vi "Robot_Main-backup.vi"() -> ()   [LabVIEW 2013]
uses:
  PolarCoordTdef.ctl
  StopTDef.ctl
  GainsTDef.ctl
  Support VIs/setpointCluster.ctl
  <vilib>/robotics/Starter Kit/2.0/9632 Host Interface/NI_Robotics_Starter Kit Host_9632_2.0.lvclass
  Support VIs/robotStop.vi
  Support VIs/gainsGlobalBot.vi
  Support VIs/setpointsGlobal.vi
  <vilib>/robotics/Starter Kit/Host Interface/NI_Robotics_Starter Kit Host.lvclass
panel:
  out "Kd-Arg":dbl
  out "Kc-Arg":dbl
  out "Kd-Mod":dbl
  out "Kc-Mod":dbl
  out "Modulus Setpoint Read":dbl
  out "Argument Setpoint Read":dbl
  out "Mod":dbl
  out "Arg":dbl
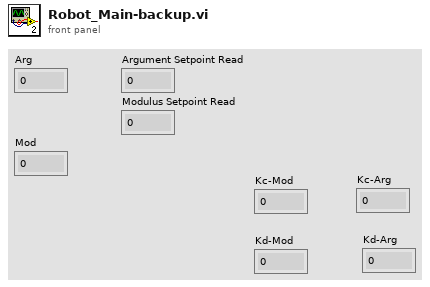
[diagram p1: front panel]
types:
  T1 = typedef "PolarCoordTdef.ctl" = cluster{"Argument":dbl, "Modulus":dbl, "trackedState":bool}
  T2 = typedef "StopTDef.ctl" = cluster{"stop":bool}
  T3 = typedef "GainsTDef.ctl" = cluster{"Kc-Modulus":dbl, "Kd-Modulus":dbl, "Kc-Argument":dbl, "Kd-Argument":dbl}
  T4 = typedef "setpointCluster.ctl" = cluster{"Modulus Setpoint":dbl, "Argument Setpoint":dbl}
  T5 = typedef "Messages.ctl" = cluster{"message data":variant, "message type":enum16{"Stop", "PolarCoordinates", "Gains", "Setpoints"}}
  T6 = cluster{"Kc-Modulus":dbl, "Kd-Modulus":dbl, "Kc-Argument":dbl, "Kd-Argument":dbl}
  T7 = enum16{"Stop", "PolarCoordinates", "Gains", "Setpoints"}
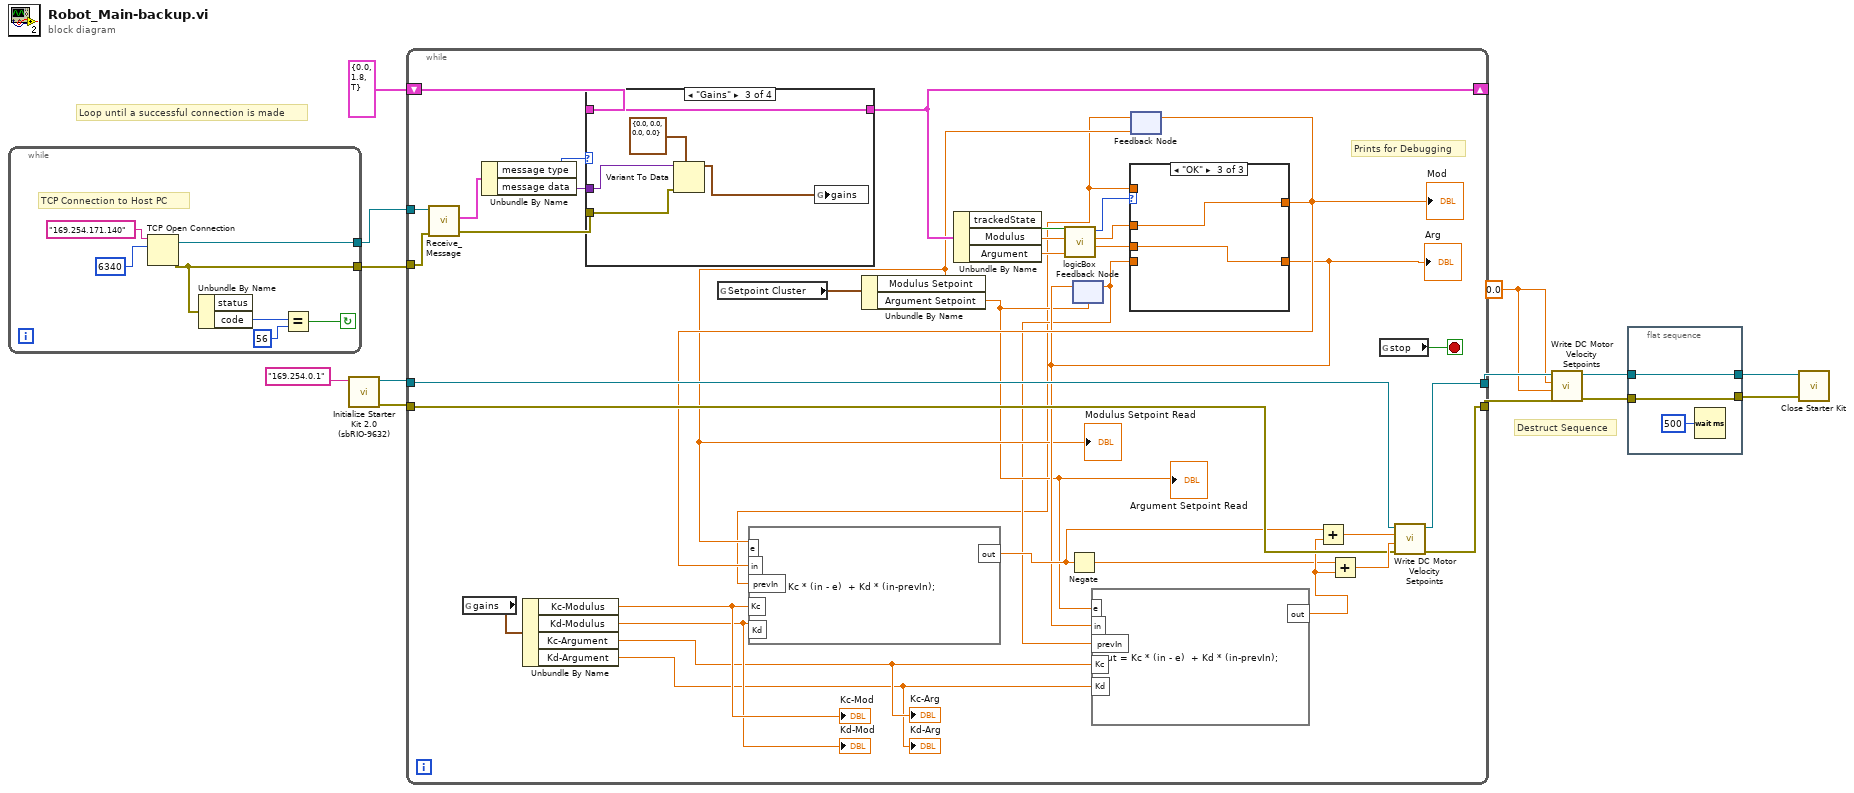
[diagram p0: block diagram]
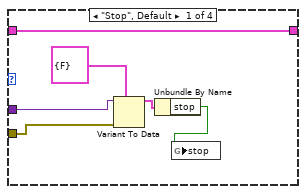
[diagram p2: hidden frame]
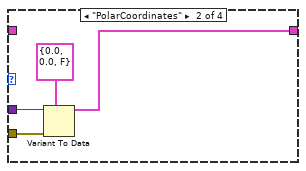
[diagram p3: hidden frame]
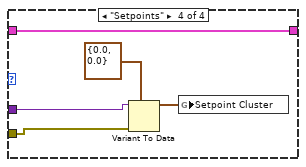
[diagram p4: hidden frame]
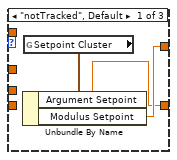
[diagram p5: hidden frame]
diagram:
  w9 = 0.0
  # "Loop until a successful connection is made"
  # "Destruct Sequence"
  n1 = while {
    tunnel: [w20] -> w2
    tunnel: [w17] -> w3
    stop <- w14 continue-if-true
    # "TCP Connection to Host PC"
    n2 = TCP Open Connection(address="169.254.171.140", remote port or service name=u16 6340) -> (connection ID=w20:refnum<k5>, error out=w17:errorcluster)  [unwired: 3 in]
    n3 = Unbundle By Name(w17) -> ("code"=w16:i32)  [unwired: 1 out]
    n4 = Equal?(x=w16, y=56) -> (x = y?=w14:bool)
  }
  n5 = call <vilib>:"Initialize Starter Kit 2.0 (sbRIO-9632).vi"("IP address (\"\")"="169.254.0.1" ("IP address (\"\")")) -> ("error out"=w12:errorcluster, "FPGA starter kit host 2.0 out"=w13:refnum<class "NI_Robotics_Starter Kit Host_9632_2.0.lvclass">)  [unwired: 9 in]
  n6 = while {
    tunnel: w13 -> [w54]
    tunnel: w12 -> [w53]
    tunnel: w3 -> [w42]
    tunnel: [w52] -> w11
    tunnel: [w51] -> w10
    tunnel: w2 -> [w43]
    shift-right: [w39] -> _
    shift-left: T1 {"Argument"=0.0, "Modulus"=1.8, "trackedState"=TRUE} ("Polar Coord") -> [w38]
    stop <- w41 stop-if-true
    # "Prints for Debugging"
    n7 = call "Receive_Message.vi"("error in (no error)"=w42, "connection ID IN"=w43) -> ("error out (no error)"=w44:errorcluster, "msg OUT"=w47:T5)  [unwired: 7 in, 1 out]
    n8 = global read "gainsGlobalBot.vi" "gains"() -> (w40:T6)
    n9 = Unbundle By Name(w47) -> ("message type"=w46:T7, "message data"=w45:variant)
    n10 = Unbundle By Name(w40) -> ("Kc-Modulus"=w24:dbl, "Kd-Modulus"=w23:dbl, "Kc-Argument"=w22:dbl, "Kd-Argument"=w21:dbl)
    "Kc-Mod" <- w24
    "Kd-Mod" <- w23
    "Kc-Arg" <- w22
    "Kd-Arg" <- w21
    n11 = case shown="\"Gains\"" w46 {
      tunnel: w45 -> [w61 w65 w70 w75]
      tunnel: w44 -> [w60 w64 w69 w74]
      tunnel: [w57 w63 w67 w72] -> w39
      tunnel: w38 -> [w57 _ w67 w72]
      frame "Stop", Default {
        n12 = Variant To Data(error in=w60, type=T2 {"stop"=FALSE}, Variant=w61) -> (data=w59:T2)  [unwired: 1 out]
        n13 = Unbundle By Name(w59) -> ("stop"=w58:bool)
        n14 = global write "robotStop.vi" "stop"(w58) -> ()
      }
      frame "PolarCoordinates" {
        n15 = Variant To Data(error in=w64, type=T1 {"Argument"=0.0, "Modulus"=0.0, "trackedState"=FALSE} ("Polar Coord"), Variant=w65) -> (data=w63:T1)  [unwired: 1 out]
      }
      frame "Gains" {
        n16 = Variant To Data(error in=w69, type=T3 {"Kc-Modulus"=0.0, "Kd-Modulus"=0.0, "Kc-Argument"=0.0, "Kd-Argument"=0.0} ("GainsCluster"), Variant=w70) -> (data=w68:T3)  [unwired: 1 out]
        n17 = global write "gainsGlobalBot.vi" "gains"(w68) -> ()
      }
      frame "Setpoints" {
        n18 = Variant To Data(error in=w74, type=T4 {"Modulus Setpoint"=0.0, "Argument Setpoint"=0.0} ("Setpoint Cluster"), Variant=w75) -> (data=w73:T4)  [unwired: 1 out]
        n19 = global write "setpointsGlobal.vi" "Setpoint Cluster"(w73) -> ()
      }
    }
    n20 = global read "setpointsGlobal.vi" "Setpoint Cluster"() -> (w29:T4)
    n21 = Unbundle By Name(w29) -> ("Modulus Setpoint"=w28:dbl, "Argument Setpoint"=w27:dbl)
    "Argument Setpoint Read" <- w27
    "Modulus Setpoint Read" <- w28
    n22 = Unbundle By Name(w39) -> ("trackedState"=w37:bool, "Modulus"=w36:dbl, "Argument"=w35:dbl)
    n23 = call "logicBox.vi"("Arg"=w35, "Mod"=w36, "TrackState"=w37) -> ("Arg"=w32:dbl, "Mod"=w33:dbl, "State"=w34:enum16{"notTracked", "NullMessage", "OK"})  [unwired: 6 in]
    n24 = feedback #1(w27) -> (w26:dbl)
    n25 = feedback #2(w28) -> (w25:dbl)
    n26 = case shown="\"OK\"" w34 {
      tunnel: [w77 w80 w82] -> w30
      tunnel: [w78 w81 w83] -> w31
      tunnel: w33 -> [_ _ w83]
      tunnel: w32 -> [_ _ w82]
      tunnel: w25 -> [_ w81 _]
      tunnel: w26 -> [_ w80 _]
      frame "notTracked", Default {
        n27 = global read "setpointsGlobal.vi" "Setpoint Cluster"() -> (w79:T4)
        n28 = Unbundle By Name(w79) -> ("Argument Setpoint"=w77:dbl, "Modulus Setpoint"=w78:dbl)
      }
      frame "NullMessage" {
      }
      frame "OK" {
      }
    }
    "Arg" <- w30
    "Mod" <- w31
    n29 = formula code="out = Kc * (in - e)  + Kd * (in-prevIn);"("e"=w28, "in"=w31, "prevIn"=w25, "Kc"=w24, "Kd"=w23) -> ("out"=w48:dbl)
    n30 = Negate(x=w48) -> (-x=w49:dbl)
    n31 = feedback-in #1(w30) -> ()
    n32 = formula code="out = Kc * (in - e)  + Kd * (in-prevIn);"("e"=w27, "in"=w30, "prevIn"=w26, "Kc"=w22, "Kd"=w21) -> ("out"=w50:dbl)
    n33 = feedback-in #2(w31) -> ()
    n34 = Add(x=w48, y=w50) -> (x+y=w56:dbl)
    n35 = Add(x=w49, y=w50) -> (x+y=w55:dbl)
    n36 = global read "robotStop.vi" "stop"() -> (w41:bool)
    n37 = call <vilib>:"Write DC Motor Velocity Setpoints.vi"("error in (no error)"=w53, "right motor ccw velocity (rad/s)"=w55, "left motor ccw velocity (rad/s)"=w56, "starter kit host in"=w54) -> ("error out"=w51:errorcluster, "starter kit host out"=w52:refnum<class "NI_Robotics_Starter Kit Host_9632_2.0.lvclass">)  [unwired: 6 in]
  }
  n38 = call <vilib>:"Write DC Motor Velocity Setpoints.vi"("error in (no error)"=w10, "right motor ccw velocity (rad/s)"=w9, "left motor ccw velocity (rad/s)"=w9, "starter kit host in"=w11) -> ("error out"=w7:errorcluster, "starter kit host out"=w8:refnum<class "NI_Robotics_Starter Kit Host_9632_2.0.lvclass">)  [unwired: 6 in]
  n39 = flat-sequence {
    tunnel: w8 -> [w85]
    tunnel: w7 -> [w84]
    tunnel: [w85] -> w6
    tunnel: [w84] -> w5
    frame #0 {
      n40 = Wait (ms)(milliseconds to wait=u32 500) -> ()  [unwired: 1 out]
    }
  }
  n41 = call-dynamic "Close Starter Kit.vi"("error in (no error)"=w5, "starter kit host in"=w6) -> ()  [unwired: 9 in, 1 out]
